vi "_Topmost UI Ref.vi"(8 "error in (no error)":errorcluster) -> (0 "error out":errorcluster, 3 "VI out":refnum<vi>)   [LabVIEW 2014, in "UI_ProgressDlg.lvlib" / "UI_ProgressDlg.lvclass"]
uses:
  UI_ProgressDlg.lvclass
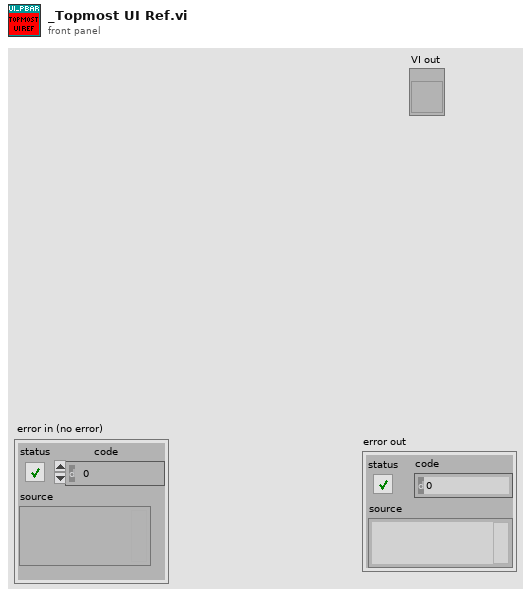
[diagram p1: front panel]
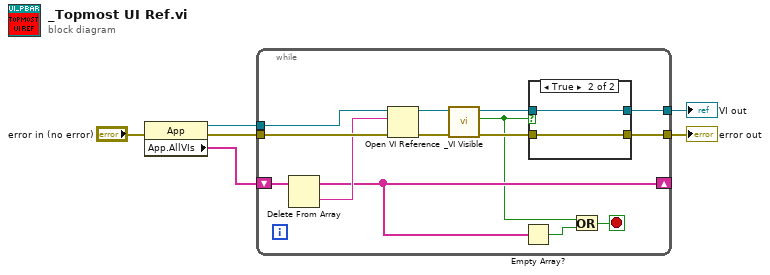
[diagram p0: block diagram]
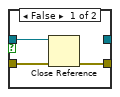
[diagram p2: hidden frame]
diagram:
  n1 = property class="App"(error in="error in (no error)") -> (reference out=w4:refnum<vi>, error out=w6:errorcluster, "App.AllVIs"=w5:string[])  [unwired: 1 in]
  n2 = while {
    tunnel: w6 -> [w18]
    tunnel: w4 -> [w15]
    shift-right: [w10] -> _
    shift-left: w5 -> [w17]
    tunnel: [w9] -> w3
    tunnel: [w7] -> w1
    stop <- w11 stop-if-true
    n3 = Delete From Array(array=w17) -> (deleted portion=w16:string, array with subset deleted=w10:string[])  [unwired: 2 in]
    n4 = Open VI Reference(application reference (local)=w15, vi path=w16, error in (no error)=w18) -> (vi reference=w20:refnum<vi>, error out=w13:errorcluster)  [unwired: 3 in]
    n5 = call "_VI Visible.vi"("error in (no error)"=w13, "VI in"=w20) -> ("error out"=w12:errorcluster, "visible"=w8:bool, "VI out"=w19:refnum<vi>)  [unwired: 7 in]
    n6 = Empty Array?(array=w10) -> (empty?=w14:bool)
    n7 = case shown="True" w8 {
      tunnel: w19 -> [w23 w24]
      tunnel: w12 -> [w22 w25]
      tunnel: [w21 w25] -> w9
      tunnel: [_ w24] -> w7
      frame False {
        n8 = Close Reference(reference=w23, error in (no error)=w22) -> (error out=w21:errorcluster)
      }
      frame True {
      }
    }
    n9 = Or(x=w8, y=w14) -> (x .or. y?=w11:bool)
  }
  "error out" <- w3
  "VI out" <- w1
